vi "Main.vi"(11 "Module Admin":refnum<class "Delacor_lib_QMH_Module Admin.lvclass">) -> ()   [LabVIEW 2019, in "Menu Launcher Module.lvlib"]
doc: "This template is based off of the Queued Message Handler design pattern and the Queued Message Handler project template that ships with LabVIEW.\n\nThe main difference is that the queue is private to this module and communication between modules is performed via Broadcast and Request events.\n\nRequest events are wrapped in public API methods and are handled in the Event Handling Loop (EHL) of this VI. Any module can register for Broadcast events sent by this module. The EHL generates messages based on user interface actions.\n\nThe Message Handling Loop (MHL) processes messages generated by the EHL, or by other messages. The messages are string values, so new messages can be added easily to the Message Cases case structure in the MHL. Each message cluster can also provide an optional value for Message Data, which is a variant that can be converted to whatever message-specific data is required.\n_____\nBased on Delacor QMH Project Template 5.0.0.82."
uses:
  Menu Launcher Module.lvlib
  <vilib>/Delacor/Delacor QMH/Libraries/Module Admin_class/Delacor_lib_QMH_Module Admin.lvclass
  Module Data--cluster.ctl
  Utility/Controls/Menu_Configuration.ctl
  <vilib>/Delacor/Delacor QMH/Libraries/Message Queue_class/Delacor_lib_QMH_Message Queue.lvclass/Delacor_lib_QMH_Message Queue.ctl
  Stop Argument--cluster.ctl
  <vilib>/Delacor/Delacor QMH/Libraries/Module Admin_class/Delacor_lib_QMH_Module Admin.lvclass/Delacor_lib_QMH_Module Admin.ctl
  Init Menu Configuration Argument--cluster.ctl
  Init Menu Argument--cluster.ctl
  Change Menu Configure Argument--cluster.ctl
  Launch Menu Argument--cluster.ctl
  Close Menu Argument--cluster.ctl
  <vilib>/Utility/miscctls.llb/LVPointTypeDef.ctl
  <vilib>/Delacor/Delacor QMH/Libraries/Message Queue_class/Delacor_lib_QMH_Enqueue Message (Single).vi
  <vilib>/Delacor/Delacor QMH/Libraries/Module Admin_class/Delacor_lib_QMH_Get External Launch.vi
  <vilib>/Utility/error.llb/Error Cluster From Error Code.vi
  <vilib>/ErrorRing/Error Ring.xnode
  <vilib>/Delacor/Delacor QMH/Libraries/Message Queue_class/Delacor_lib_QMH_Message Queue.lvclass
  Menu Module/Menu Module.lvlib
panel:
  in  "Simulate MHL Error":bool
  in  "Simulate EHL Error":bool
  out "error out":errorcluster
  out "Status":string
  # "Other QMH Modules communicate with this Module via its Public API (wrappers for its Request Events).\n\nThis Module communicates with other Modules via its Broadcast Events.\nAny module that wants to get these messages, just registers for this module's Broadcast events."
  # "This template is for the Delacor Modified Queued Message Handler design pattern.\n\nSee the block diagram for more information on how to use this template."
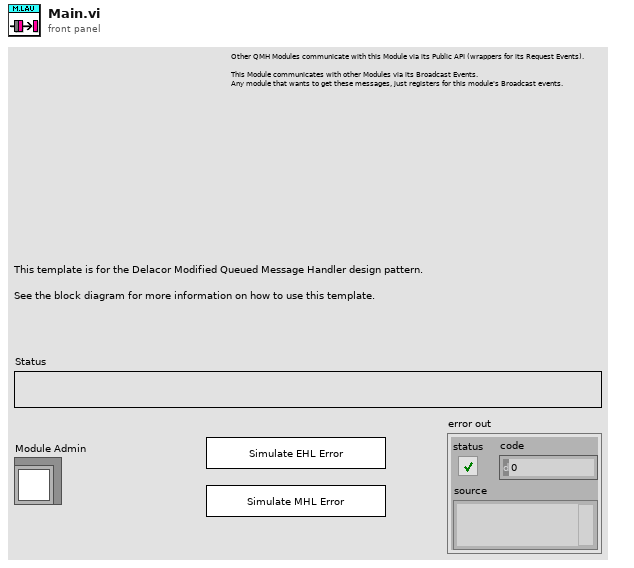
[diagram p1: front panel]
types:
  T1 = typedef "Menu Launcher Module.lvlib/Request Events--cluster.ctl" = cluster{"Stop Module":refnum<user-event>, "Show Panel":refnum<user-event>, "Hide Panel":refnum<user-event>, "Get Module Execution Status":refnum<user-event>, "Show Diagram":refnum<user-event>, "Init Menu Configuration":refnum<user-event>, "Init Menu":refnum<user-event>, "Change Menu Configure":refnum<user-event>, "Launch Menu":refnum<user-event>, "Close Menu":refnum<user-event>}
  T2 = typedef "Menu Module.lvlib/Broadcast Events--cluster.ctl" = cluster{"Module Did Init":refnum<user-event>, "Status Updated":refnum<user-event>, "Error Reported":refnum<user-event>, "Module Did Stop":refnum<user-event>, "Update Module Execution Status":refnum<user-event>, "Button Pressed":refnum<user-event>}
  T3 = typedef "Menu Launcher Module.lvlib/Module Data--cluster.ctl" = cluster{"Status":string, "Menu_Configuration":T4, "Root Module ID":i32}
  T4 = typedef "Menu_Configuration.ctl" = cluster{"Button_Label_Color":u32, "Button_Color_On":u32, "Button_Color_Off":u32, "Panel_Color":u32, "Extend_Sub_Menu_Icon":path, "Root_Menu_Data":cluster{"Button_Icon":path, "Button_Label":string, "Sub_Menu_Data":cluster{"Button_Icon":path, "Button_Label":string, "Child_Menu_Data":cluster{"Button_Icon":path, "Button_Label":string}[]}[]}[]}
  T5 = enum32{"invalid lock state", "Not Locked", "Locked (No Password)", "Password-protected"}
  T6 = typedef "Menu Launcher Module.lvlib/Stop Argument--cluster.ctl" = cluster{"Origin":string, "Exit via Stop Module Req?":bool, "Wait for Module to stop?":bool}
  T7 = typedef "Menu Launcher Module.lvlib/Init Menu Configuration Argument--cluster.ctl" = cluster{"Menu File Path":path}
  T8 = typedef "Menu Launcher Module.lvlib/Init Menu Argument--cluster.ctl" = cluster{"Menu_Configuration":T4, "Module ID":i32}
  T9 = typedef "Menu Launcher Module.lvlib/Change Menu Configure Argument--cluster.ctl" = cluster{"Menu Configuration Path":path}
  T10 = typedef "Menu Launcher Module.lvlib/Launch Menu Argument--cluster.ctl" = cluster{"Position":cluster{"Top":i16, "Left":i16}}
  T11 = typedef "Menu Launcher Module.lvlib/Close Menu Argument--cluster.ctl" = cluster{"Boolean":bool}
  T12 = typedef "LVPointTypeDef.ctl" = cluster{"Horizontal":i16, "Vertical":i16}
  T13 = enum32{"Invalid", "Standard", "Closed", "Hidden", "Minimized", "Maximized"}
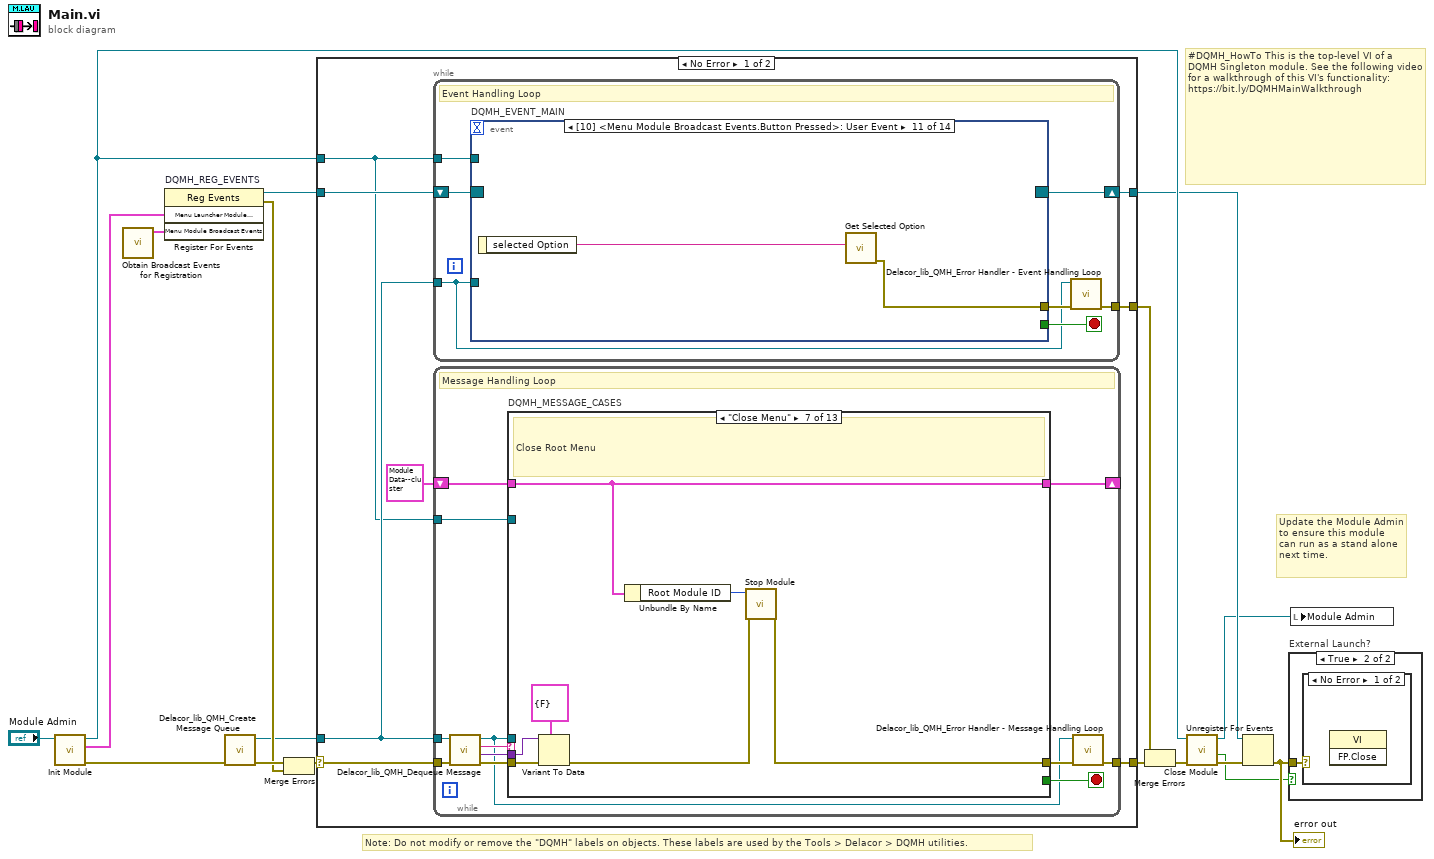
[diagram p0: block diagram]
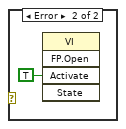
[diagram p3: hidden frame]
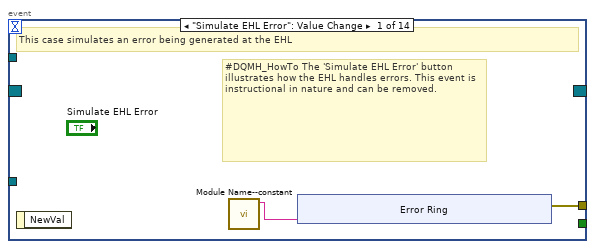
[diagram p4: hidden frame]
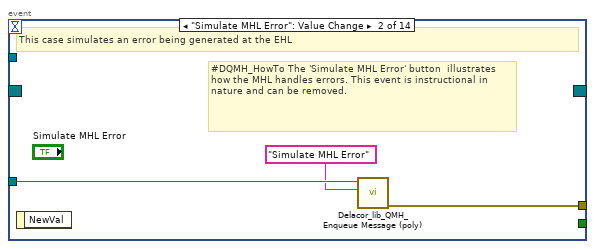
[diagram p5: hidden frame]
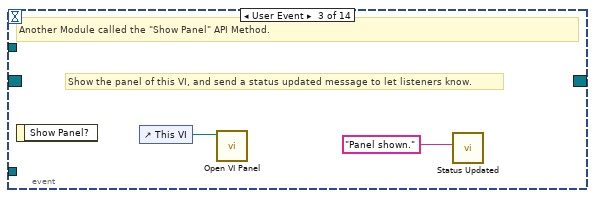
[diagram p6: hidden frame]
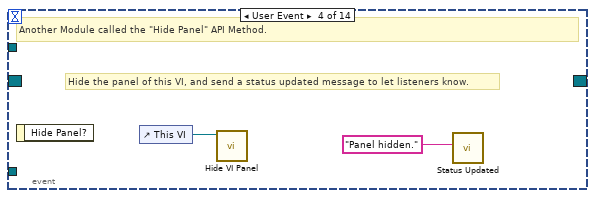
[diagram p7: hidden frame]
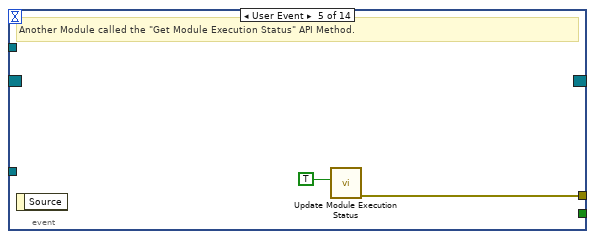
[diagram p8: hidden frame]
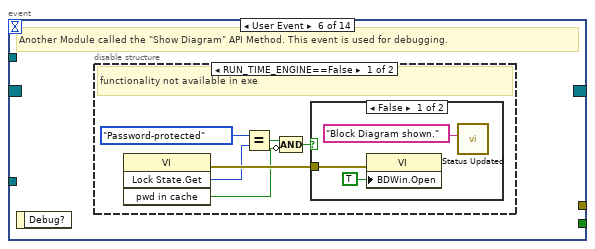
[diagram p9: hidden frame]
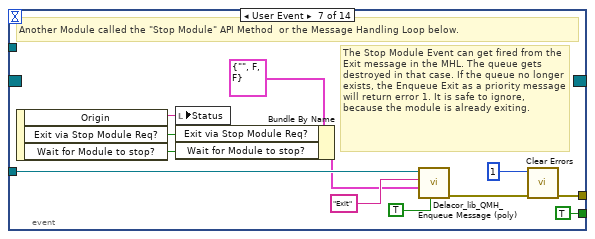
[diagram p12: hidden frame]
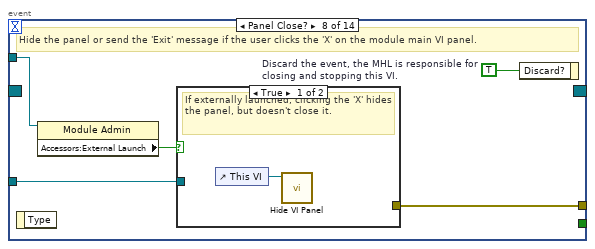
[diagram p13: hidden frame]
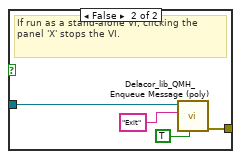
[diagram p14: hidden frame]
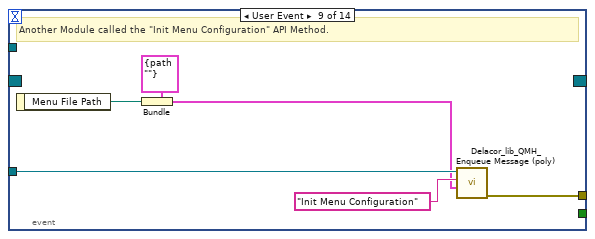
[diagram p15: hidden frame]
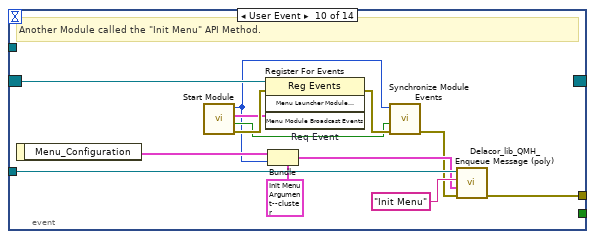
[diagram p16: hidden frame]
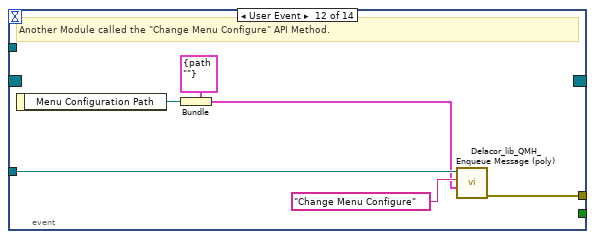
[diagram p17: hidden frame]
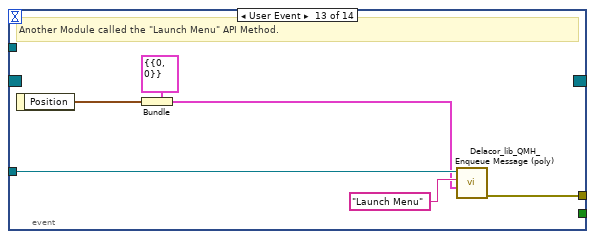
[diagram p18: hidden frame]
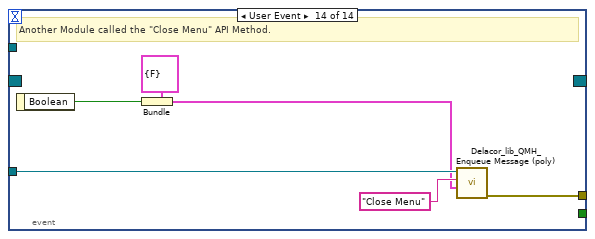
[diagram p19: hidden frame]
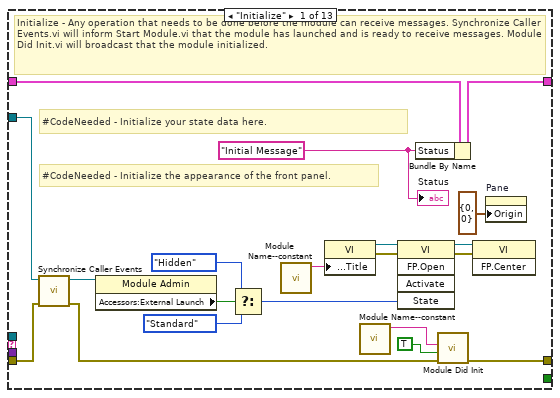
[diagram p20: hidden frame]
diagram:
  # "#DQMH_HowTo This is the top-level VI of a DQMH Singleton module. See the following video for a walkthrough of this VI's functionality: https://bit.ly/DQMHMainWalkthrough"
  # "Note: Do not modify or remove the \"DQMH\" labels on objects. These labels are used by the Tools > Delacor > DQMH utilities."
  # "Update the Module Admin to ensure this module can run as a stand alone next time."
  n1 = call "Init Module.vi"("Singleton Module Admin in"="Module Admin") -> ("error out"=w17:errorcluster, "Menu Launcher Module Request Events"=w6:T1, "Singleton Module Admin out"=w9:refnum<class "Delacor_lib_QMH_Module Admin.lvclass">)  [unwired: 8 in]
  n2 = call "Obtain Broadcast Events for Registration.vi"() -> ("Menu Module Broadcast Events"=w1:T2)  [unwired: 9 in, 2 out]
  n3 = register-events "DQMH_REG_EVENTS"(w6, w1) -> (reference out=w7:refnum<event-registration>, error out=w10:errorcluster)  [unwired: 2 in]
  n4 = call <vilib>:"Delacor_lib_QMH_Create Message Queue.vi"("error in"=w17) -> ("error out"=w12:errorcluster, "Message Queue"=w5:refnum<class "Delacor_lib_QMH_Message Queue.lvclass">)  [unwired: 9 in]
  n5 = Merge Errors(w12, w10) -> (w11:errorcluster)
  n6 = case shown="No Error" w11 {
    selector: w11 -> [w24 w280]
    tunnel: [w26 w279] -> w18
    tunnel: [w23 w285] -> w8
    tunnel: w7 -> [w21 w285]
    tunnel: w5 -> [w20 w278]
    tunnel: [w25 _] -> w15
    tunnel: w9 -> [w19 w281]
    frame No Error {
      n7 = while {
        tunnel: w20 -> [w27]
        shift-right: [w30] -> w23
        shift-left: w21 -> [w31]
        tunnel: [w32] -> w25
        tunnel: w19 -> [w28]
        stop <- w29 stop-if-true
        # "Event Handling Loop"
        n8 = event "DQMH_EVENT_MAIN" shown="[10] <Menu Module Broadcast Events.Button Pressed>: User Event" {
          selector: w31 -> [_ _ _ _ _ _ _ _ _ w92 _ _ _ _]
          dyn-events: [_ _ _ _ _ _ _ _ _ _ _ _ _ _] -> w30
          timeout: _ -> [_ _ _ _ _ _ _ _ _ _ _ _ _ _]
          tunnel: [_ _ _ _ _ _ TRUE ("Discard?") _ _ _ _ _ _ _] -> w29
          tunnel: w27 -> [_ w44 _ _ _ _ w68 w75 w88 w101 _ w109 w115 w121]
          tunnel: [w35 w45 _ _ w51 _ w71 w77 w83 w96 w102 w104 w110 w116] -> w33
          tunnel: w28 -> [_ _ _ _ _ _ _ w74 _ _ _ _ _ _]
          event "Simulate EHL Error": Value Change {
            # "#DQMH_HowTo The 'Simulate EHL Error' button  illustrates how the EHL handles errors. This event is instructional in nature and can be removed."
            # "This case simulates an error being generated at the EHL"
            n9 = event-data() -> ()  [unwired: 1 in, 1 out]
            n10 = call "Module Name--constant.vi"() -> ("Module Name"=w34:string)  [unwired: 11 in]
            n11 = xnode "Error Ring"("parameter 0"=w34) -> ("error out"=w35:errorcluster)
          }
          event "Simulate MHL Error": Value Change {
            # "#DQMH_HowTo The 'Simulate MHL Error' button  illustrates how the MHL handles errors. This event is instructional in nature and can be removed."
            # "This case simulates an error being generated at the EHL"
            n12 = event-data() -> ()  [unwired: 1 in, 1 out]
            n13 = call-poly <vilib>:"Delacor_lib_QMH_Enqueue Message (poly).vi"("Message"="Simulate MHL Error", "Message Queue in"=w44) -> ("error out"=w45:errorcluster)  [unwired: 8 in, 1 out]
          }
          event User Event {
            # "Show the panel of this VI, and send a status updated message to let listeners know."
            # "Another Module called the \"Show Panel\" API Method."
            n14 = event-data() -> ()  [unwired: 1 in, 1 out]
            n15 = control-ref of="This VI"() -> (w47:refnum<vi>)
            n16 = call "Open VI Panel.vi"("VI"=w47) -> ()  [unwired: 10 in, 1 out]
            n17 = call "Status Updated.vi"("Status"="Panel shown." ("format string")) -> ()  [unwired: 10 in, 1 out]
          }
          event User Event {
            # "Hide the panel of this VI, and send a status updated message to let listeners know."
            # "Another Module called the \"Hide Panel\" API Method."
            n18 = event-data() -> ()  [unwired: 1 in, 1 out]
            n19 = control-ref of="This VI"() -> (w49:refnum<vi>)
            n20 = call "Hide VI Panel.vi"("VI"=w49) -> ()  [unwired: 10 in, 1 out]
            n21 = call "Status Updated.vi"("Status"="Panel hidden." ("format string")) -> ()  [unwired: 10 in, 1 out]
          }
          event User Event {
            # "Another Module called the \"Get Module Execution Status\" API Method."
            n22 = event-data() -> ()  [unwired: 1 in, 1 out]
            n23 = call "Update Module Execution Status.vi"("Running?"=TRUE) -> ("error out"=w51:errorcluster)  [unwired: 10 in]
          }
          event User Event {
            # "Another Module called the \"Show Diagram\" API Method. This event is used for debugging."
            n24 = event-data() -> ()  [unwired: 1 in, 1 out]
            n25 = disable-structure shown="RUN_TIME_ENGINE==False" {
              frame condition #0 (active) {
                # "functionality not available in exe"
                n26 = invoke class="VI" method="Lock State.Get"() -> (error out=w57:errorcluster, "Get Lock State"=w56:T5, "pwd in cache"=w53:bool)  [unwired: 4 in, 1 out]
                n27 = Equal?(x=T5."Password-protected", y=w56) -> (x = y?=w54:bool)
                n28 = Compound Arithmetic op=AND(w54, invert w53) -> (w52:bool)
                n29 = case shown="False" w52 {
                  tunnel: w57 -> [w60 _]
                  frame False {
                    n30 = property class="VI"(error in=w60, "BDWin.Open"=TRUE ("Block Diagram Window:Open")) -> ()  [unwired: 1 in, 2 out]
                    n31 = call "Status Updated.vi"("Status"="Block Diagram shown." ("format string")) -> ()  [unwired: 10 in, 1 out]
                  }
                  frame True {
                    # "Password-protected VI, and the password is not in the cache. Do not show the diagram."
                  }
                }
              }
              frame condition #1 {
              }
            }
          }
          event User Event {
            # "The Stop Module Event can get fired from the Exit message in the MHL. The queue gets destroyed in that case. If the queue no longer exists, the Enqueue Exit as a priority message will return error 1. It is safe to ignore, because the module is already exiting."
            # "Another Module called the \"Stop Module\" API Method  or the Message Handling Loop below."
            n32 = event-data() -> ("Origin"=w67:string, "Exit via Stop Module Req?"=w63:bool, "Wait for Module to stop?"=w62:bool)  [unwired: 1 in]
            n33 = local write "Status"(w67) -> ()
            n34 = Bundle By Name(cluster=T6 {"Origin"="", "Exit via Stop Module Req?"=FALSE, "Wait for Module to stop?"=FALSE} ("Stop Argument"), "Exit via Stop Module Req?"=w63, "Wait for Module to stop?"=w62) -> (w61:T6)
            n35 = call-poly <vilib>:"Delacor_lib_QMH_Enqueue Message (poly).vi"("Priority Message? (F)"=TRUE, "Message Data"=w61, "Message"="Exit", "Message Queue in"=w68) -> ("error out"=w72:errorcluster)  [unwired: 6 in, 1 out]
            n36 = call <vilib>:"Clear Errors.vi"("error in (no error)"=w72, "specific error code to clear (0: all)"=1) -> ("error out"=w71:errorcluster)  [unwired: 4 in, 1 out]
          }
          event Panel Close? {
            w76 = TRUE  # Discard the event, the MHL is responsible for closing and stopping this VI.
            # "Hide the panel or send the 'Exit' message if the user clicks the 'X' on the module main VI panel."
            n37 = event-data() -> ()  [unwired: 1 in, 1 out]
            n38 = property class="Module Admin"(reference=w74) -> ("Accessors:External Launch"=w73:bool)  [unwired: 1 in, 2 out]
            n39 = case shown="True" w73 {
              tunnel: w75 -> [_ w81]
              tunnel: [_ w82] -> w77
              frame True {
                # "If externally launched, clicking the 'X' hides the panel, but doesn't close it."
                n40 = control-ref of="This VI"() -> (w78:refnum<vi>)
                n41 = call "Hide VI Panel.vi"("VI"=w78) -> ()  [unwired: 10 in, 1 out]
              }
              frame False {
                # "If run as a stand-alone VI, clicking the panel 'X' stops the VI."
                n42 = call-poly <vilib>:"Delacor_lib_QMH_Enqueue Message (poly).vi"("Priority Message? (F)"=TRUE, "Message"="Exit", "Message Queue in"=w81) -> ("error out"=w82:errorcluster)  [unwired: 7 in, 1 out]
              }
            }
            n43 = event-data("Discard?"=w76) -> ()  [unwired: 1 in, 1 out]
          }
          event User Event {
            # "Another Module called the \"Init Menu Configuration\" API Method."
            n44 = event-data() -> ("Menu File Path"=w84:path)  [unwired: 1 in]
            n45 = Bundle(cluster=T7 {"Menu File Path"=path ""} ("Init Menu Configuration Argument"), "Menu File Path"=w84) -> (w85:T7)
            n46 = call-poly <vilib>:"Delacor_lib_QMH_Enqueue Message (poly).vi"("Message Data"=w85, "Message"="Init Menu Configuration", "Message Queue in"=w88) -> ("error out"=w83:errorcluster)  [unwired: 7 in, 1 out]
          }
          event User Event {
            # "Another Module called the \"Init Menu\" API Method."
            n47 = event-data() -> ("Menu_Configuration"=w97:T4)  [unwired: 1 in]
            n48 = call "Start Module.vi"() -> ("error out"=w95:errorcluster, "Wait for Event Sync?"=w91:bool, "Menu Module Broadcast Events"=w94:T2, "Module ID"=w90:i32)  [unwired: 8 in]
            n49 = register-events "Req Event"(reference=w92, error in=w95, w94) -> (error out=w93:errorcluster)  [unwired: 1 in, 1 out]
            n50 = Bundle(cluster=T8 {"Menu_Configuration"={"Button_Label_Color"=2344, "Button_Color_On"=5654, "Button_Color_Off"=2344, "Panel_Color"=2344, "Extend_Sub_Menu_Icon"=path "C:/Users/SyncSols-4/Desktop/Icon/Accept-icon.png", "Root_Menu_Data"=[{"Button_Icon"=path "C:/Users/SyncSols-4/Desktop/Icon/Accept-icon.png", "Button_Label"="Test", "Sub_Menu_Data"=[{"Button_Icon"=path "C:/Users/SyncSols-4/Desktop/Icon/floppy-icon.png", "Button_Label"="Save", "Child_Menu_Data"=[]}, {"Button_Icon"=path "C:/Users/SyncSols-4/Desktop/Icon/folder-icon1.png", "Button_Label"="Folder", "Child_Menu_Data"=[]}, {"Button_Icon"=path "C:/Users/SyncSols-4/Desktop/Icon/delete-icon.png", "Button_Label"="Delete", "Child_Menu_Data"=[{"Button_Icon"=path "C:/Users/SyncSols-4/Desktop/Icon/add-icon.png", "Button_Label"="Add"}, {"Button_Icon"=path "C:/Users/SyncSols-4/Desktop/Icon/Stop-red-icon.png", "Button_Label"="Stop"}]}]}, {"Button_Icon"=path "C:/Users/SyncSols-4/Desktop/Icon/add-key-icon.png", "Button_Label"="Key", "Sub_Menu_Data"=[]}, {"Button_Icon"=path "C:/Users/SyncSols-4/Desktop/Icon/Categories-preferences-system-icon.png", "Button_Label"="Setting", "Sub_Menu_Data"=[]}]}, "Module ID"=0} ("Init Menu Argument"), "Menu_Configuration"=w97, "Module ID"=w90) -> (w98:T8)
            n51 = call "Synchronize Module Events.vi"("error in (no error)"=w93, "Wait for Event Sync?"=w91, "Module ID"=w90) -> ("error out"=w89:errorcluster)  [unwired: 7 in, 1 out]
            n52 = call-poly <vilib>:"Delacor_lib_QMH_Enqueue Message (poly).vi"("error in"=w89, "Message Data"=w98, "Message"="Init Menu", "Message Queue in"=w101) -> ("error out"=w96:errorcluster)  [unwired: 6 in, 1 out]
          }
          event User Event {
            n53 = event-data() -> ("selected Option"=w103:string)  [unwired: 1 in]
            n54 = call "Get Selected Option.vi"("Selected Options"=w103) -> ("error out"=w102:errorcluster)  [unwired: 10 in]
          }
          event User Event {
            # "Another Module called the \"Change Menu Configure\" API Method."
            n55 = event-data() -> ("Menu Configuration Path"=w105:path)  [unwired: 1 in]
            n56 = Bundle(cluster=T9 {"Menu Configuration Path"=path ""} ("Change Menu Configure Argument"), "Menu Configuration Path"=w105) -> (w106:T9)
            n57 = call-poly <vilib>:"Delacor_lib_QMH_Enqueue Message (poly).vi"("Message Data"=w106, "Message"="Change Menu Configure", "Message Queue in"=w109) -> ("error out"=w104:errorcluster)  [unwired: 7 in, 1 out]
          }
          event User Event {
            # "Another Module called the \"Launch Menu\" API Method."
            n58 = event-data() -> ("Position"=w111:cluster{"Top":i16, "Left":i16})  [unwired: 1 in]
            n59 = Bundle(cluster=T10 {"Position"={"Top"=0, "Left"=0}} ("Launch Menu Argument"), "Position"=w111) -> (w112:T10)
            n60 = call-poly <vilib>:"Delacor_lib_QMH_Enqueue Message (poly).vi"("Message Data"=w112, "Message"="Launch Menu", "Message Queue in"=w115) -> ("error out"=w110:errorcluster)  [unwired: 7 in, 1 out]
          }
          event User Event {
            # "Another Module called the \"Close Menu\" API Method."
            n61 = event-data() -> ("Boolean"=w117:bool)  [unwired: 1 in]
            n62 = Bundle(cluster=T11 {"Boolean"=FALSE} ("Close Menu Argument"), "Boolean"=w117) -> (w118:T11)
            n63 = call-poly <vilib>:"Delacor_lib_QMH_Enqueue Message (poly).vi"("Message Data"=w118, "Message"="Close Menu", "Message Queue in"=w121) -> ("error out"=w116:errorcluster)  [unwired: 7 in, 1 out]
          }
        }
        n64 = call-dynamic "Delacor_lib_QMH_Error Handler - Event Handling Loop.vi"("error in"=w33, "Message Queue in"=w27) -> ("dup error in"=w32:errorcluster)  [unwired: 8 in, 1 out]
      }
      n65 = while {
        tunnel: w20 -> [w124]
        shift-right: [w128] -> _
        shift-left: T3 {"Status"="", "Menu_Configuration"={"Button_Label_Color"=2344, "Button_Color_On"=5654, "Button_Color_Off"=2344, "Panel_Color"=2344, "Extend_Sub_Menu_Icon"=path "C:/Users/SyncSols-4/Desktop/Icon/Accept-icon.png", "Root_Menu_Data"=[{"Button_Icon"=path "C:/Users/SyncSols-4/Desktop/Icon/Accept-icon.png", "Button_Label"="Test", "Sub_Menu_Data"=[{"Button_Icon"=path "C:/Users/SyncSols-4/Desktop/Icon/floppy-icon.png", "Button_Label"="Save", "Child_Menu_Data"=[]}, {"Button_Icon"=path "C:/Users/SyncSols-4/Desktop/Icon/folder-icon1.png", "Button_Label"="Folder", "Child_Menu_Data"=[]}, {"Button_Icon"=path "C:/Users/SyncSols-4/Desktop/Icon/delete-icon.png", "Button_Label"="Delete", "Child_Menu_Data"=[{"Button_Icon"=path "C:/Users/SyncSols-4/Desktop/Icon/add-icon.png", "Button_Label"="Add"}, {"Button_Icon"=path "C:/Users/SyncSols-4/Desktop/Icon/Stop-red-icon.png", "Button_Label"="Stop"}]}]}, {"Button_Icon"=path "C:/Users/SyncSols-4/Desktop/Icon/add-key-icon.png", "Button_Label"="Key", "Sub_Menu_Data"=[]}, {"Button_Icon"=path "C:/Users/SyncSols-4/Desktop/Icon/Categories-preferences-system-icon.png", "Button_Label"="Setting", "Sub_Menu_Data"=[]}]}, "Root Module ID"=0} ("Data Cluster") -> [w129]
        tunnel: w24 -> [w132]
        tunnel: [w130] -> w26
        tunnel: w19 -> [w122]
        stop <- w127 stop-if-true
        # "Message Handling Loop"
        n66 = call-dynamic "Delacor_lib_QMH_Dequeue Message.vi"("error in"=w132, "Message Queue in"=w124) -> ("error out"=w131:errorcluster, "Message Data"=w125:variant, "Message"=w126:string, "Message Queue out"=w123:refnum<class "Delacor_lib_QMH_Message Queue.lvclass">)  [unwired: 6 in]
        n67 = case "DQMH_MESSAGE_CASES" shown="\"Close Menu\"" w126 {
          selector: w126 -> [_ _ _ _ _ _ _ _ _ _ _ _ w265]
          tunnel: w123 -> [_ _ _ _ _ _ _ _ _ _ w235 w257 _]
          tunnel: w131 -> [w151 w155 w170 w181 w198 w207 w214 w217 w219 w224 w242 w263 w267]
          tunnel: [w149 w155 w158 w176 w184 w199 w208 w216 w219 w223 w238 w260 w268] -> w133
          tunnel: w129 -> [w140 w154 w169 w172 w187 w202 w211 w215 w218 w221 w237 w256 w266]
          tunnel: [w139 w154 w157 w174 w183 w202 w211 w215 w218 w221 w237 w256 w266] -> w128
          tunnel: [_ _ _ _ _ _ _ _ _ _ _ w255 _] -> w127
          tunnel: w125 -> [_ _ w168 w180 w197 w206 w213 _ _ _ w236 w254 _]
          tunnel: w122 -> [w141 _ _ _ _ _ _ _ _ _ w234 w249 _]
          frame "Initialize" {
            w134 = "Initial Message" ("Initial Message")
            # "#CodeNeeded - Initialize the appearance of the front panel."
            # "#CodeNeeded - Initialize your state data here."
            # "Initialize - Any operation that needs to be done before the module can receive messages. Synchronize Caller Events.vi will inform Start Module.vi that the module has launched and is ready to receive messages. Module Did Init.vi will broadcast that the module initialized."
            n68 = call "Synchronize Caller Events.vi"("error in (no error)"=w151, "Singleton Module Admin in"=w141) -> ("error out"=w150:errorcluster, "Singleton Module Admin out"=w136:refnum<class "Delacor_lib_QMH_Module Admin.lvclass">)  [unwired: 8 in]
            n69 = property class="Module Admin"(reference=w136) -> ("Accessors:External Launch"=w145:bool)  [unwired: 1 in, 2 out]
            n70 = Select(t=T13."Hidden" ("State"), s=w145, f=T13."Standard" ("State")) -> (s? t:f=w142:T13)
            n71 = call "Module Name--constant.vi"() -> ("Module Name"=w148:string)  [unwired: 11 in]
            n72 = property class="VI"("Front Panel.Title"=w148) -> (reference out=w147:refnum<vi>, error out=w153:errorcluster)  [unwired: 2 in]
            n73 = call "Module Name--constant.vi"() -> ("Module Name"=w137:string)  [unwired: 11 in]
            n74 = invoke class="VI" method="FP.Open"(reference=w147, error in=w153, "State"=w142) -> (reference out=w146:refnum<vi>, error out=w152:errorcluster)  [unwired: 2 in, 3 out]
            n75 = Bundle By Name(cluster=w140, "Status"=w134) -> (w139:T3)
            n76 = call "Module Did Init.vi"("error in (no error)"=w150, "Initialized?"=TRUE, "Origin"=w137) -> ("error out"=w149:errorcluster)  [unwired: 8 in]
            n77 = invoke class="VI" method="FP.Center"(reference=w146, error in=w152) -> ()  [unwired: 1 in, 3 out]
            n78 = property on="Pane" class="Pane"("Origin"=T12 {"Horizontal"=0, "Vertical"=0}) -> ()  [unwired: 2 in, 2 out]
            "Status" <- w134
          }
          frame "--- Module Specific ---" {
            # "Separator -- The following cases handle messages specific to this Module."
          }
          frame "Init Menu Configuration" {
            w161 = T4 {"Button_Label_Color"=2344, "Button_Color_On"=5654, "Button_Color_Off"=2344, "Panel_Color"=2344, "Extend_Sub_Menu_Icon"=path "C:/Users/SyncSols-4/Desktop/Icon/Accept-icon.png", "Root_Menu_Data"=[{"Button_Icon"=path "C:/Users/SyncSols-4/Desktop/Icon/Accept-icon.png", "Button_Label"="Test", "Sub_Menu_Data"=[{"Button_Icon"=path "C:/Users/SyncSols-4/Desktop/Icon/floppy-icon.png", "Button_Label"="Save", "Child_Menu_Data"=[]}, {"Button_Icon"=path "C:/Users/SyncSols-4/Desktop/Icon/folder-icon1.png", "Button_Label"="Folder", "Child_Menu_Data"=[]}, {"Button_Icon"=path "C:/Users/SyncSols-4/Desktop/Icon/delete-icon.png", "Button_Label"="Delete", "Child_Menu_Data"=[{"Button_Icon"=path "C:/Users/SyncSols-4/Desktop/Icon/add-icon.png", "Button_Label"="Add"}, {"Button_Icon"=path "C:/Users/SyncSols-4/Desktop/Icon/Stop-red-icon.png", "Button_Label"="Stop"}]}]}, {"Button_Icon"=path "C:/Users/SyncSols-4/Desktop/Icon/add-key-icon.png", "Button_Label"="Key", "Sub_Menu_Data"=[]}, {"Button_Icon"=path "C:/Users/SyncSols-4/Desktop/Icon/Categories-preferences-system-icon.png", "Button_Label"="Setting", "Sub_Menu_Data"=[]}]} ("Menu_Configuration")
            # "This will Read and Init the Menu Configuration"
            n79 = Variant To Data(error in=w170, type=T7 {"Menu File Path"=path ""} ("Init Menu Configuration Argument"), Variant=w168) -> (data=w166:T7, error out=w159:errorcluster)
            n80 = Unbundle By Name(w166) -> ("Menu File Path"=w165:path)
            n81 = Read from Text File(file (use dialog)=w165, error in=w159) -> (text=w164:string, error out=w160:errorcluster)  [unwired: 2 in, 2 out]
            n82 = call <vilib>:"Easy Parse XML__JKI EasyXML.vi"("error in (no error)"=w160, "LabVIEW Data (Type)"=w161, "XML String"=w164) -> ("error out"=w163:errorcluster, "LabVIEW Data"=w162:variant)  [unwired: 7 in]
            n83 = Variant To Data(error in=w163, type=w161, Variant=w162) -> (data=w156:T4, error out=w158:errorcluster)
            n84 = Bundle By Name(cluster=w169, "Menu_Configuration"=w156) -> (w157:T3)
          }
          frame "Init Menu" {
            # "Init Menu With the Menu File"
            n85 = Variant To Data(error in=w181, type=T8 {"Menu_Configuration"={"Button_Label_Color"=2344, "Button_Color_On"=5654, "Button_Color_Off"=2344, "Panel_Color"=2344, "Extend_Sub_Menu_Icon"=path "C:/Users/SyncSols-4/Desktop/Icon/Accept-icon.png", "Root_Menu_Data"=[{"Button_Icon"=path "C:/Users/SyncSols-4/Desktop/Icon/Accept-icon.png", "Button_Label"="Test", "Sub_Menu_Data"=[{"Button_Icon"=path "C:/Users/SyncSols-4/Desktop/Icon/floppy-icon.png", "Button_Label"="Save", "Child_Menu_Data"=[]}, {"Button_Icon"=path "C:/Users/SyncSols-4/Desktop/Icon/folder-icon1.png", "Button_Label"="Folder", "Child_Menu_Data"=[]}, {"Button_Icon"=path "C:/Users/SyncSols-4/Desktop/Icon/delete-icon.png", "Button_Label"="Delete", "Child_Menu_Data"=[{"Button_Icon"=path "C:/Users/SyncSols-4/Desktop/Icon/add-icon.png", "Button_Label"="Add"}, {"Button_Icon"=path "C:/Users/SyncSols-4/Desktop/Icon/Stop-red-icon.png", "Button_Label"="Stop"}]}]}, {"Button_Icon"=path "C:/Users/SyncSols-4/Desktop/Icon/add-key-icon.png", "Button_Label"="Key", "Sub_Menu_Data"=[]}, {"Button_Icon"=path "C:/Users/SyncSols-4/Desktop/Icon/Categories-preferences-system-icon.png", "Button_Label"="Setting", "Sub_Menu_Data"=[]}]}, "Module ID"=0} ("Init Menu Argument"), Variant=w180) -> (data=w178:T8, error out=w177:errorcluster)
            n86 = Unbundle By Name(w172) -> ("Menu_Configuration"=w171:T4)
            n87 = Unbundle By Name(w178) -> ("Module ID"=w173:i32)
            n88 = call "Init Menu.vi"("Menu Type"=enum16{"Root", "Sub", "Child"}."Root", "error in (no error)"=w177, "Menu_Configuration"=w171, "Module ID"=w173) -> ("error out"=w176:errorcluster)  [unwired: 7 in]
            n89 = Bundle By Name(cluster=w172, "Root Module ID"=w173) -> (w174:T3)
          }
          frame "Change Menu Configure" {
            w191 = T4 {"Button_Label_Color"=2344, "Button_Color_On"=5654, "Button_Color_Off"=2344, "Panel_Color"=2344, "Extend_Sub_Menu_Icon"=path "C:/Users/SyncSols-4/Desktop/Icon/Accept-icon.png", "Root_Menu_Data"=[{"Button_Icon"=path "C:/Users/SyncSols-4/Desktop/Icon/Accept-icon.png", "Button_Label"="Test", "Sub_Menu_Data"=[{"Button_Icon"=path "C:/Users/SyncSols-4/Desktop/Icon/floppy-icon.png", "Button_Label"="Save", "Child_Menu_Data"=[]}, {"Button_Icon"=path "C:/Users/SyncSols-4/Desktop/Icon/folder-icon1.png", "Button_Label"="Folder", "Child_Menu_Data"=[]}, {"Button_Icon"=path "C:/Users/SyncSols-4/Desktop/Icon/delete-icon.png", "Button_Label"="Delete", "Child_Menu_Data"=[{"Button_Icon"=path "C:/Users/SyncSols-4/Desktop/Icon/add-icon.png", "Button_Label"="Add"}, {"Button_Icon"=path "C:/Users/SyncSols-4/Desktop/Icon/Stop-red-icon.png", "Button_Label"="Stop"}]}]}, {"Button_Icon"=path "C:/Users/SyncSols-4/Desktop/Icon/add-key-icon.png", "Button_Label"="Key", "Sub_Menu_Data"=[]}, {"Button_Icon"=path "C:/Users/SyncSols-4/Desktop/Icon/Categories-preferences-system-icon.png", "Button_Label"="Setting", "Sub_Menu_Data"=[]}]} ("Menu_Configuration")
            # "Change the Menu Configuration File"
            n90 = Variant To Data(error in=w198, type=T9 {"Menu Configuration Path"=path ""} ("Change Menu Configure Argument"), Variant=w197) -> (data=w195:T9, error out=w185:errorcluster)
            n91 = Unbundle By Name(w195) -> ("Menu Configuration Path"=w189:path)
            n92 = Unbundle By Name(w187) -> ("Root Module ID"=w186:i32)
            n93 = Read from Text File(file (use dialog)=w189, error in=w185) -> (text=w194:string, error out=w190:errorcluster)  [unwired: 2 in, 2 out]
            n94 = call <vilib>:"Easy Parse XML__JKI EasyXML.vi"("error in (no error)"=w190, "LabVIEW Data (Type)"=w191, "XML String"=w194) -> ("error out"=w193:errorcluster, "LabVIEW Data"=w192:variant)  [unwired: 7 in]
            n95 = Variant To Data(error in=w193, type=w191, Variant=w192) -> (data=w182:T4, error out=w188:errorcluster)
            n96 = Bundle By Name(cluster=w187, "Menu_Configuration"=w182) -> (w183:T3)
            n97 = call "Init Menu.vi"("error in (no error)"=w188, "Menu_Configuration"=w182, "Module ID"=w186) -> ("error out"=w184:errorcluster)  [unwired: 8 in]
          }
          frame "Launch Menu" {
            # "Launch the Root Menu"
            n98 = Variant To Data(error in=w207, type=T10 {"Position"={"Top"=0, "Left"=0}} ("Launch Menu Argument"), Variant=w206) -> (data=w204:T10, error out=w200:errorcluster)
            n99 = Unbundle By Name(w202) -> ("Root Module ID"=w201:i32)
            n100 = Unbundle By Name(w204) -> ("Position"=w203:cluster{"Top":i16, "Left":i16})
            n101 = call "Resize the Panel.vi"("error in (no error)"=w200, "Position"=w203, "Module ID"=w201) -> ("error out"=w199:errorcluster)  [unwired: 8 in]
          }
          frame "Close Menu" {
            # "Close Root Menu"
            n102 = Variant To Data(error in=w214, type=T11 {"Boolean"=FALSE} ("Close Menu Argument"), Variant=w213) -> (error out=w209:errorcluster)  [unwired: 1 out]
            n103 = Unbundle By Name(w211) -> ("Root Module ID"=w210:i32)
            n104 = call "Stop Module.vi"("error in (no error)"=w209, "Module ID"=w210) -> ("error out"=w208:errorcluster)  [unwired: 9 in]
          }
          frame "---Copy This Frame---" {
            # "Duplicate this frame when creating new messages.  Change this comment in the duplicated frame to describe this message."
            n105 = Merge Errors(w217) -> (w216:errorcluster)
          }
          frame "--- Exit and Error Handling---" {
            # "Separator - The following cases handle errors and exit messages."
          }
          frame "Simulate MHL Error" {
            # "#DQMH_HowTo The 'Simulate MHL Error' button  illustrates how the MHL handles errors. This event is instructional in nature and can be removed."
            # "Simulate an error occurring at the MHL"
            n106 = call "Module Name--constant.vi"() -> ("Module Name"=w220:string)  [unwired: 11 in]
            n107 = xnode "Error Ring"("parameter 0"=w220) -> ("error out"=w222:errorcluster)
            n108 = Merge Errors(w224, w222) -> (w223:errorcluster)
          }
          frame "Error" {
            # "#CodeRecommended - If you ever change the name of this \"Error\" message, you'll need to update the name in the Check Loop Error.vi as well."
            # "#CodeRecommended - If the module is running in standalone mode (External Launch = FALSE), this code will pop up an error dialog and call the 'Exit' message if an error occurs. Add more fine-grained error handling here."
            # "Error - Check the error message data and respond accordingly. This message is sent by the \"Error Handler\" VIs at the end of each loop in this application."
            n109 = property class="Module Admin"(reference=w234) -> ("Accessors:External Launch"=w233:bool)  [unwired: 1 in, 2 out]
            n110 = Variant To Data(error in=w242, type=errorcluster {"status"=FALSE, "code"=0, "source"=""} ("error constant"), Variant=w236) -> (data=w243:errorcluster, error out=w240:errorcluster)
            n111 = call "Module Name--constant.vi"() -> ("Module Name"=w232:string)  [unwired: 11 in]
            n112 = call "Error Reported.vi"("Additional Information"=w232, "Error"=w243) -> ()  [unwired: 9 in, 1 out]
            n113 = case shown="False" w233 {
              tunnel: [w248 _] -> w239
              tunnel: w235 -> [w246 _]
              tunnel: w243 -> [w247 _]
              frame False {
                # "If the module is running standalone, then pop up an error dialog and call the \"Exit\" message."
                n114 = call <vilib>:"Simple Error Handler.vi"("error in (no error)"=w247) -> ()  [unwired: 4 in, 5 out]
                n115 = call-poly <vilib>:"Delacor_lib_QMH_Enqueue Message (poly).vi"("Priority Message? (F)"=TRUE, "Message"="Exit", "Message Queue in"=w246) -> ("error out"=w248:errorcluster)  [unwired: 7 in, 1 out]
              }
              frame True {
                # "If the module was launched externally, calling the Error Reported broadcast VI is the only action performed by the \"Error\" message. The module's caller can then process the error appropriately."
              }
            }
            n116 = Merge Errors(w240, w239) -> (w238:errorcluster)
            n117 = local write "error out"(w238) -> ()
          }
          frame "Exit" {
            w253 = 91  # 91: not all Exit messages will have an argument
            w255 = TRUE  # Stop the VI
            # "Release the message queue reference"
            # "#CodeNeeded - Add any required cleanup code here"
            # "Exit - Exit the application."
            n118 = Variant To Data(error in=w263, type=T6 {"Origin"="", "Exit via Stop Module Req?"=FALSE, "Wait for Module to stop?"=FALSE} ("Stop Argument"), Variant=w254) -> (data=w251:T6, error out=w259:errorcluster)
            n119 = call <vilib>:"Clear Errors.vi"("error in (no error)"=w259, "specific error code to clear (0: all)"=w253) -> ("error out"=w262:errorcluster)  [unwired: 4 in, 1 out]
            n120 = control-ref of="This VI"() -> (w250:refnum<vi>)
            n121 = call-dynamic "Delacor_lib_QMH_Release Message Queue.vi"("error in"=w262, "Message Queue"=w257) -> ("error out"=w261:errorcluster)  [unwired: 9 in]
            n122 = call "Handle Exit.vi"("Stop Argument"=w251, "Admin in"=w249, "VI reference"=w250) -> ("error out"=w258:errorcluster)  [unwired: 7 in, 1 out]
            n123 = Merge Errors(w261, w258) -> (w260:errorcluster)
          }
          frame Default {
            # "'Default' case only runs if there is a message that isn't defined in any of the other cases.  Output a programming error."
            n124 = call "Module Name--constant.vi"() -> ("Module Name"=w264:string)  [unwired: 11 in]
            n125 = xnode "Error Ring"("parameter 0"=w265, "parameter 1"=w264) -> ("error out"=w269:errorcluster)
            n126 = Merge Errors(w267, w269) -> (w268:errorcluster)
          }
        }
        n127 = call-dynamic "Delacor_lib_QMH_Error Handler - Message Handling Loop.vi"("error in"=w133, "Message Queue in"=w123) -> ("dup error in"=w130:errorcluster)  [unwired: 8 in, 1 out]
      }
    }
    frame Error {
      # "Synchronize Caller Events.vi will inform Start Module.vi that the module has launched and will let the code calling Start Module.vi register for broadcasts and would permit the caller receive the broadcast that an error occurred at launch time."
      n128 = call-dynamic "Delacor_lib_QMH_Release Message Queue.vi"("error in"=w280, "Message Queue"=w278) -> ("error out"=w279:errorcluster)  [unwired: 9 in]
      n129 = call "Synchronize Caller Events.vi"("Singleton Module Admin in"=w281) -> ("error out"=w286:errorcluster)  [unwired: 9 in, 1 out]
      n130 = call "Module Name--constant.vi"() -> ("Module Name"=w284:string)  [unwired: 11 in]
      n131 = Format Into String(format string="An error occurred during initialization. %s is no longer running.", w284) -> (resulting string=w282:string)  [unwired: 2 in, 1 out]
      n132 = Merge Errors(w279, w286) -> (w287:errorcluster)
      n133 = call "Error Reported.vi"("Additional Information"=w282, "Error"=w287) -> ()  [unwired: 9 in, 1 out]
    }
  }
  n134 = Merge Errors(w15, w18) -> (w14:errorcluster)
  n135 = call "Close Module.vi"("error in (no error)"=w14, "Module Admin in"=w9) -> ("error out"=w16:errorcluster, "External Launch"=w2:bool, "Module Admin out"=w3:refnum<class "Delacor_lib_QMH_Module Admin.lvclass">)  [unwired: 7 in]
  n136 = Unregister For Events(event registration refnum=w8, error in=w16) -> (error out=w13:errorcluster)
  "error out" <- w13
  n137 = case "External Launch?" shown="True" w2 {
    tunnel: w13 -> [_ w288]
    frame False {
    }
    frame True {
      n138 = case shown="No Error" w288 {
        frame No Error {
          n139 = invoke class="VI" method="FP.Close"() -> ()  [unwired: 3 in, 3 out]
        }
        frame Error {
          n140 = invoke class="VI" method="FP.Open"("Activate"=TRUE ("Activate?")) -> ()  [unwired: 4 in, 5 out]
        }
      }
    }
  }
  n141 = local write "Module Admin"(w3) -> ()
